vi "discoverCANinterface_backup.vi"() -> (2 "FPGA VI":refnum<k20>, 3 "FC":refnum<k21>, 4 "Converter":refnum<k21>, 5 "CANdiscovered":bool)   [LabVIEW 2021]
uses:
  <vilib>/rvi/interface/nirviOpenFPGA/nirviOpenFPGA.xnode
  <vilib>/rvi/interface/nirviMethod/nirviMethod.xnode
  <vilib>/FPGAPlugInAG/Dynamic/niLvFpga_Run_Dynamic.vi
  FPGA Bitfiles/HydrogenAgent_FPGATarget2_RMSacq_UgSXIwAP2ko.lvbitx
  RMSacq.vi
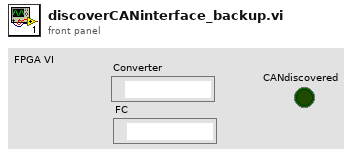
[diagram p1: front panel]
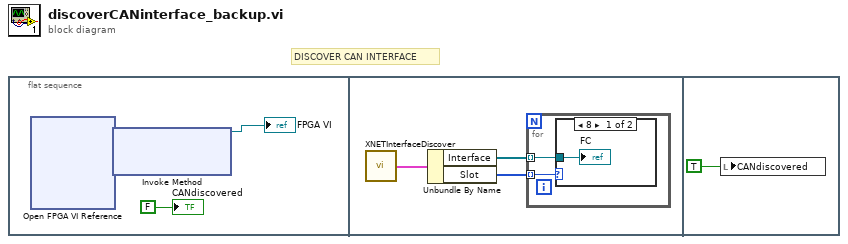
[diagram p0: block diagram]
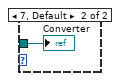
[diagram p2: hidden frame]
diagram:
  # "DISCOVER CAN INTERFACE"
  n1 = flat-sequence {
    frame #0 {
      n2 = xnode "Open FPGA VI Reference"() -> ("FPGA VI Reference Out"=w3:refnum<k20>, "error out"=w4:errorcluster)  [unwired: 2 in]
      n3 = xnode "Invoke Method"("FPGA VI Reference In"=w3, "error in"=w4) -> ("FPGA VI Reference Out"=→"FPGA VI":refnum<k20>)  [unwired: 1 in, 1 out]
      "CANdiscovered" <- FALSE
    }
    frame #1 {
      n4 = call "XNETInterfaceDiscover.vi"() -> ("CAN"=w5:cluster{"Interface":refnum<k21>[], "Slot":u32[]})  [unwired: 1 in]
      n5 = Unbundle By Name(w5) -> ("Interface"=w6:refnum<k21>[], "Slot"=w7:u32[])
      n6 = for {
        tunnel: w7 -> [w9] mode=indexing
        tunnel: w6 -> [w8] mode=indexing
        n7 = case shown="8" w9 {
          tunnel: w8 -> [w10 w11]
          frame 8 {
            "FC" <- w10
          }
          frame 7, Default {
            "Converter" <- w11
          }
        }
      }
    }
    frame #2 {
      n8 = local write "CANdiscovered"(TRUE) -> ()
    }
  }
